vi "setUp.vi"(8 "error in (no error)":errorcluster, 11 "reference in":refnum<class "Test Network Stream Nested Endpoint.lvclass">) -> (0 "error out":errorcluster, 3 "reference out":refnum<class "Test Network Stream Nested Endpoint.lvclass">)   [LabVIEW 2020, in "Test Network Stream Nested Endpoint.lvclass"]
doc: "setUp runs prior to the test method during test execution. Use this method to initialize any object data required by your tests."
uses:
  Test Network Stream Nested Endpoint.lvclass
  <vilib>/addons/_JKI Toolkits/VI Tester/TestCase.llb/TestCase.lvclass
  <vilib>/ActorFramework/Actor/Actor.lvclass
  <vilib>/ActorFramework/Message Queue/Message Queue.lvclass
  Source/Ciphers/AES/AES.lvclass
  Source/Ciphers/AES/Ton Plomp Encryption/AES-Modes.ctl
  Source/Ciphers/AES/Ton Plomp Encryption/Encryption.lvlib
  Source/Protocols/Network Stream Strategy/Network Stream Initiator/Network Stream Initiator.lvclass
  Source/Nested Endpoint/Nested Endpoint/Nested Endpoint.lvclass
  Source/Network Endpoint/Network Endpoint/Network Endpoint.lvclass
  Source/Protocols/Network Stream Strategy/Netowrk Stream Listener/Network Stream Listener.lvclass
  Source/Abstract Classes/Message Stream/Message Stream.lvclass
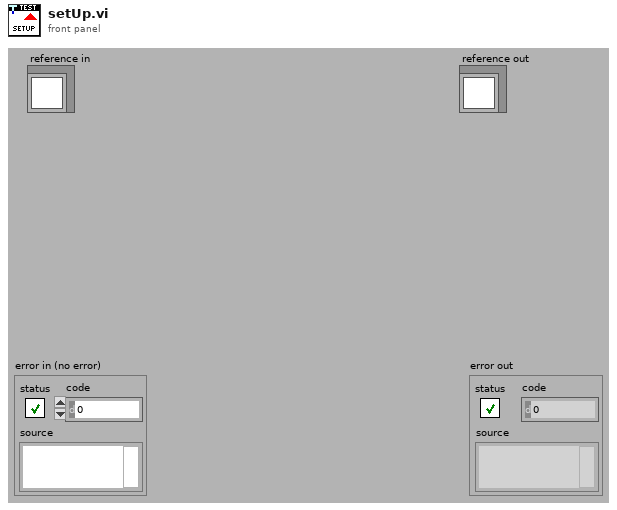
[diagram p1: front panel]
types:
  T1 = typedef "Encryption.lvlib/AES-Modes.ctl" = enum16{"ECB", "CBC", "CFB128", "OFB"}
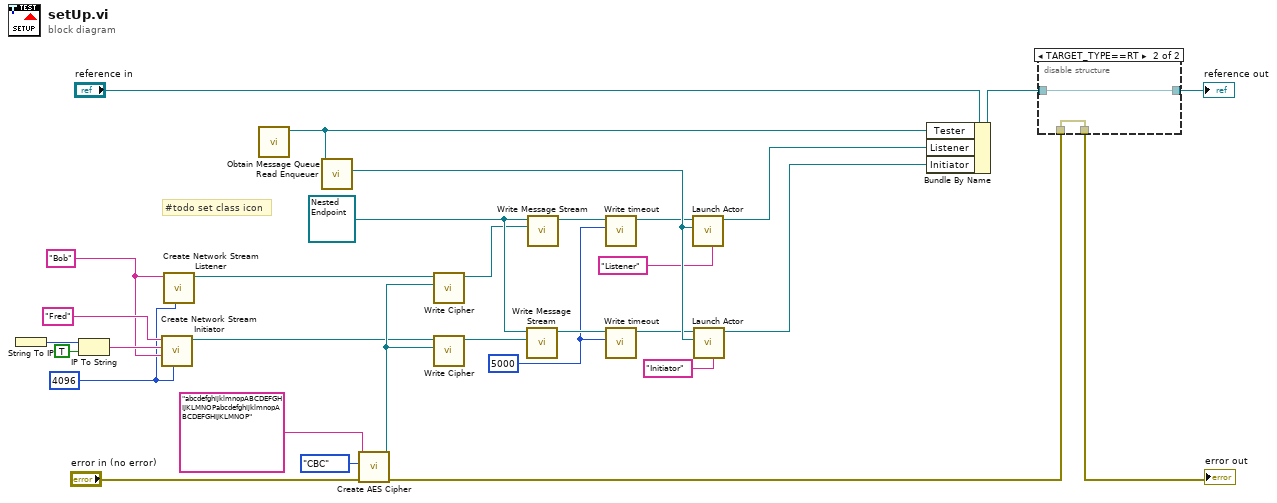
[diagram p0: block diagram]
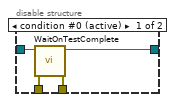
[diagram p2: hidden frame]
diagram:
  w1 = 4096 ("Buffer Size")
  w2 = "Bob" ("Name")
  w11 = 5000 ("timeout")
  w21 = refnum<class "Nested Endpoint.lvclass"> refnum ("Nested Endpoint.lvlib:Nested Endpoint.lvclass")
  # "#todo set class icon"
  n1 = String To IP() -> (0:w6:u32)  [unwired: 1 in]
  n2 = IP To String(1:TRUE ("dot notation? (F)"), 2:w6) -> (0:w5:string)
  n3 = call "Create Network Stream Initiator.vi"("Buffer Size"=w1, "Remote Name"=w2, "Remote Address"=w5, "Name"="Fred") -> ("Network Stream Initiator out"=w8:refnum<class "Network Stream Initiator.lvclass">)  [unwired: 7 in]
  n4 = call "Create Network Stream Listener.vi"("Buffer Size"=w1, "Name"=w2) -> ("Network Stream Listener"=w3:refnum<class "Network Stream Listener.lvclass">)  [unwired: 9 in]
  n5 = call <vilib>:"Obtain Message Queue.vi"() -> ("Message Queue"=w16:refnum<class "Message Queue.lvclass">)  [unwired: 10 in, 1 out]
  n6 = call <vilib>:"Read Enqueuer.vi"("Message Queue"=w16) -> ("Message Enqueuer"=w27:refnum<class "Message Enqueuer.lvclass">)  [unwired: 10 in]
  n7 = call "Create AES Cipher.vi"("error in (no error)"="error in (no error)", "Operation Mode"=AES-Modes."CBC", "Cipher Key"="abcdefghijklmnopABCDEFGHIJKLMNOPabcdefghijklmnopABCDEFGHIJKLMNOP") -> ("error out"=w23:errorcluster, "AES out"=w22:refnum<class "AES.lvclass">)  [unwired: 7 in]
  n8 = call "Write Cipher.vi"("Cipher"=w22, "Message Stream in"=w3) -> ("Message Stream out"=w20:refnum<class "Network Stream Listener.lvclass">)  [unwired: 9 in]
  n9 = call "Write Cipher.vi"("Cipher"=w22, "Message Stream in"=w8) -> ("Message Stream out"=w19:refnum<class "Network Stream Initiator.lvclass">)  [unwired: 9 in]
  n10 = call "Write Message Stream.vi"("Message Stream"=w19, "Network Endpoint in"=w21) -> ("Network Endpoint out"=w13:refnum<class "Nested Endpoint.lvclass">)  [unwired: 9 in]
  n11 = call "Write Message Stream.vi"("Message Stream"=w20, "Network Endpoint in"=w21) -> ("Network Endpoint out"=w15:refnum<class "Nested Endpoint.lvclass">)  [unwired: 9 in]
  n12 = call "Write timeout.vi"("timeout"=w11, "Network Endpoint in"=w15) -> ("Network Endpoint out"=w14:refnum<class "Nested Endpoint.lvclass">)  [unwired: 9 in]
  n13 = call "Write timeout.vi"("timeout"=w11, "Network Endpoint in"=w13) -> ("Network Endpoint out"=w12:refnum<class "Nested Endpoint.lvclass">)  [unwired: 9 in]
  n14 = call <vilib>:"Launch Actor.vi"("Debug Alias"="Listener", "Actor-to-Caller Enqueuer"=w27, "Actor"=w14) -> ("Caller-To-Actor Enqueuer"=w18:refnum<class "Message Enqueuer.lvclass">)  [unwired: 7 in, 1 out]
  n15 = call <vilib>:"Launch Actor.vi"("Debug Alias"="Initiator", "Actor-to-Caller Enqueuer"=w27, "Actor"=w12) -> ("Caller-To-Actor Enqueuer"=w17:refnum<class "Message Enqueuer.lvclass">)  [unwired: 7 in, 1 out]
  n16 = Bundle By Name(cluster="reference in", "Tester"=w16, "Listener"=w18, "Initiator"=w17) -> (w28:refnum<class "Test Network Stream Nested Endpoint.lvclass">)
  n17 = disable-structure shown="TARGET_TYPE==RT" {
    disable-tunnel: w23 -> [w35 w36]
    disable-tunnel: [w34 w36] -> w31
    disable-tunnel: [w33 w37] -> w29
    disable-tunnel: w28 -> [w32 w37]
    frame condition #0 (active) {
      n18 = call <vilib>:"WaitOnTestComplete.vi"("error in (no error)"=w35, "TestCase in"=w32) -> ("error out"=w34:errorcluster, "TestCase out"=w33:refnum<class "Test Network Stream Nested Endpoint.lvclass">)  [unwired: 8 in]
    }
    frame condition #1 {
    }
  }
  "error out" <- w31
  "reference out" <- w29
